vi "Put Row.vi"(0 "TreeNode in":refnum<class "TreeNode.lvclass">, 5 "Row data":refnum<class "Data.lvclass">, 7 "Time":i64, 9 "Size (1024)":i32=1024, 11 "error in (no error)":errorcluster) -> (4 "TreeNode out":refnum<class "TreeNode.lvclass">, 15 "error out":errorcluster)   [LabVIEW 2012, in "MDSplus.lvlib" / "TreeNode.lvclass"]
doc: "Write a single row of timestamped data."
uses:
  <vilib>/MDSplus/Classes/Data_Class/TreeNode_Class/TreeNode.lvclass
  <vilib>/MDSplus/Classes/Data_Class/Data.lvclass
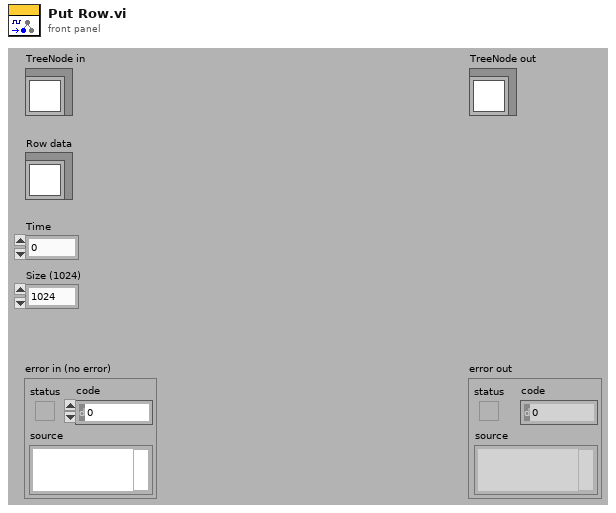
[diagram p1: front panel]
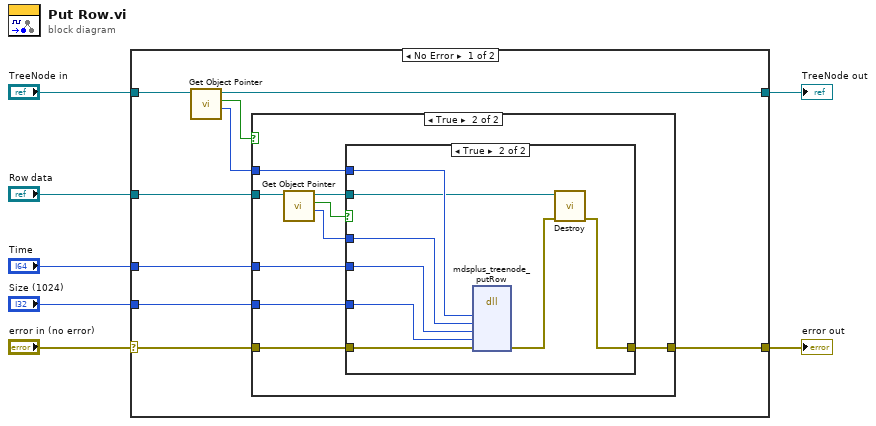
[diagram p0: block diagram]
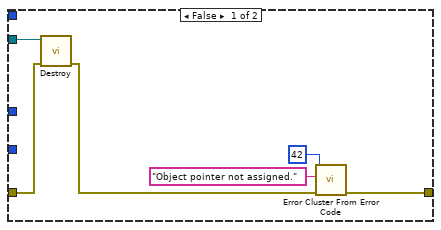
[diagram p2: hidden frame]
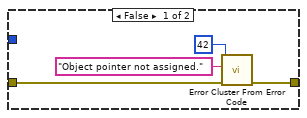
[diagram p3: hidden frame]
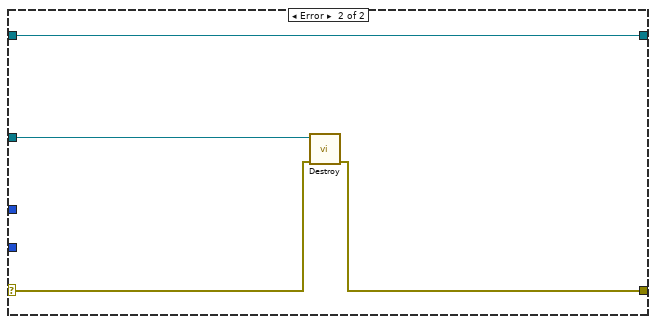
[diagram p4: hidden frame]
diagram:
  n1 = case shown="No Error" "error in (no error)" {
    selector: "error in (no error)" -> [w12 w45]
    tunnel: [w11 w44] -> w6
    tunnel: [w10 w47] -> w4
    tunnel: "TreeNode in" -> [w16 w47]
    tunnel: "Row data" -> [w15 w46]
    tunnel: "Time" -> [w9 _]
    tunnel: "Size (1024)" -> [w8 _]
    frame No Error {
      n2 = call-dynamic "Get Object Pointer.vi"("Data in"=w16) -> ("Object Pointer"=w13:i64, "Assigned object pointer?"=w14:bool, "Data out"=w10:refnum<class "TreeNode.lvclass">)  [unwired: 8 in]
      n3 = case shown="True" w14 {
        tunnel: w15 -> [w19 w31]
        tunnel: w13 -> [_ w28]
        tunnel: w12 -> [w18 w27]
        tunnel: [w20 w26] -> w11
        tunnel: w9 -> [_ w25]
        tunnel: w8 -> [_ w24]
        frame False {
          n4 = call-dynamic "Destroy.vi"("error in (no error)"=w18, "Data in"=w19) -> ("error out"=w17:errorcluster)  [unwired: 9 in]
          n5 = call <vilib>:"Error Cluster From Error Code.vi"("error in (no error)"=w17, "error message (\"\")"="Object pointer not assigned." ("error message (\"\")"), "error code (0)"=42) -> ("error out"=w20:errorcluster)  [unwired: 6 in]
        }
        frame True {
          n6 = call-dynamic "Get Object Pointer.vi"("Data in"=w31) -> ("Object Pointer"=w29:i64, "Assigned object pointer?"=w30:bool, "Data out"=w23:refnum<class "Data.lvclass">)  [unwired: 8 in]
          n7 = case shown="True" w30 {
            tunnel: w29 -> [_ w42]
            tunnel: w28 -> [_ w43]
            tunnel: w27 -> [w33 w41]
            tunnel: [w32 w36] -> w26
            tunnel: w25 -> [_ w40]
            tunnel: w24 -> [_ w39]
            tunnel: w23 -> [_ w38]
            frame False {
              n8 = call <vilib>:"Error Cluster From Error Code.vi"("error in (no error)"=w33, "error message (\"\")"="Object pointer not assigned." ("error message (\"\")"), "error code (0)"=42) -> ("error out"=w32:errorcluster)  [unwired: 6 in]
            }
            frame True {
              n9 = dll-call lib="MDSobjectsLVShr" fn="mdsplus_treenode_putRow"("lvTreeNodePtr"=w43, "lvDataPtrIn"=w42, "timeIn"=w40, "sizeIn"=w39, "error"=w41) -> ("error"=w37:errorcluster)  [unwired: 8 in, 2 out]
              n10 = call-dynamic "Destroy.vi"("error in (no error)"=w37, "Data in"=w38) -> ("error out"=w36:errorcluster)  [unwired: 9 in]
            }
          }
        }
      }
    }
    frame Error {
      n11 = call-dynamic "Destroy.vi"("error in (no error)"=w45, "Data in"=w46) -> ("error out"=w44:errorcluster)  [unwired: 9 in]
    }
  }
  "error out" <- w6
  "TreeNode out" <- w4
